vi "check out and in tracking spot null tester.vi"(0 "N spot tracker in":T1, 1 "set state?":bool, 5 "tracking state in":T2={"x state"={"pos estimate"=0.0, "v estimate"=0.0, "weighted position error sum"=0.0, "photon count"=0, "transmit tick count"=0, "axis number"=0, "px (levels^2)"=0.0, "pxv (levels^2/ticks)"=0.0, "pv (levels^2/ticks^2)"=0.0, "vel diff (levels^2/ticks^3)"=0.0, "gx"=0.0, "rtwiddle"=0.0, "photon count ch0"=0, "photon count ch1"=0, "Dx - for pos only k-f"=0.0}, "y state"={"pos estimate"=0.0, "v estimate"=0.0, "weighted position error sum"=0.0, "photon count"=0, "transmit tick count"=0, "axis number"=1, "px (levels^2)"=0.0, "pxv (levels^2/ticks)"=0.0, "pv (levels^2/ticks^2)"=0.0, "vel diff (levels^2/ticks^3)"=0.0, "gx"=0.0, "rtwiddle"=0.0, "photon count ch0"=0, "photon count ch1"=0, "Dx - for pos only k-f"=0.0}, "z state"={"pos estimate"=0.0, "v estimate"=0.0, "weighted position error sum"=0.0, "photon count"=0, "transmit tick count"=0, "axis number"=2, "px (levels^2)"=0.0, "pxv (levels^2/ticks)"=0.0, "pv (levels^2/ticks^2)"=0.0, "vel diff (levels^2/ticks^3)"=0.0, "gx"=0.0, "rtwiddle"=0.0, "photon count ch0"=0, "photon count ch1"=0, "Dx - for pos only k-f"=0.0}}, 7 "new circle":bool, 9 "permission to swap states":bool, 11 "set state value":T2={"x state"={"pos estimate"=0.0, "v estimate"=0.0, "weighted position error sum"=0.0, "photon count"=0, "transmit tick count"=0, "axis number"=0, "px (levels^2)"=0.0, "pxv (levels^2/ticks)"=0.0, "pv (levels^2/ticks^2)"=0.0, "vel diff (levels^2/ticks^3)"=0.0, "gx"=0.0, "rtwiddle"=0.0, "photon count ch0"=0, "photon count ch1"=0, "Dx - for pos only k-f"=0.0}, "y state"={"pos estimate"=0.0, "v estimate"=0.0, "weighted position error sum"=0.0, "photon count"=0, "transmit tick count"=0, "axis number"=1, "px (levels^2)"=0.0, "pxv (levels^2/ticks)"=0.0, "pv (levels^2/ticks^2)"=0.0, "vel diff (levels^2/ticks^3)"=0.0, "gx"=0.0, "rtwiddle"=0.0, "photon count ch0"=0, "photon count ch1"=0, "Dx - for pos only k-f"=0.0}, "z state"={"pos estimate"=0.0, "v estimate"=0.0, "weighted position error sum"=0.0, "photon count"=0, "transmit tick count"=0, "axis number"=2, "px (levels^2)"=0.0, "pxv (levels^2/ticks)"=0.0, "pv (levels^2/ticks^2)"=0.0, "vel diff (levels^2/ticks^3)"=0.0, "gx"=0.0, "rtwiddle"=0.0, "photon count ch0"=0, "photon count ch1"=0, "Dx - for pos only k-f"=0.0}}, 12 "state number to set":u8) -> (4 "N spot tracker out":T1, 6 "tracking state out":T2={"x state"={"pos estimate"=0.0, "v estimate"=0.0, "weighted position error sum"=0.0, "photon count"=0, "transmit tick count"=0, "axis number"=0, "px (levels^2)"=0.0, "pxv (levels^2/ticks)"=0.0, "pv (levels^2/ticks^2)"=0.0, "vel diff (levels^2/ticks^3)"=0.0, "gx"=0.0, "rtwiddle"=0.0, "photon count ch0"=0, "photon count ch1"=0, "Dx - for pos only k-f"=0.0}, "y state"={"pos estimate"=0.0, "v estimate"=0.0, "weighted position error sum"=0.0, "photon count"=0, "transmit tick count"=0, "axis number"=1, "px (levels^2)"=0.0, "pxv (levels^2/ticks)"=0.0, "pv (levels^2/ticks^2)"=0.0, "vel diff (levels^2/ticks^3)"=0.0, "gx"=0.0, "rtwiddle"=0.0, "photon count ch0"=0, "photon count ch1"=0, "Dx - for pos only k-f"=0.0}, "z state"={"pos estimate"=0.0, "v estimate"=0.0, "weighted position error sum"=0.0, "photon count"=0, "transmit tick count"=0, "axis number"=2, "px (levels^2)"=0.0, "pxv (levels^2/ticks)"=0.0, "pv (levels^2/ticks^2)"=0.0, "vel diff (levels^2/ticks^3)"=0.0, "gx"=0.0, "rtwiddle"=0.0, "photon count ch0"=0, "photon count ch1"=0, "Dx - for pos only k-f"=0.0}}, 8 "checked out state number":u8, 10 "use photons to track":bool)   [LabVIEW 2010]
uses:
  kalman 3-axis state.ctl
  integrating single axis kalman state.ctl
  kalman N spot state.ctl
panel:
  in  "tracking?":bool=TRUE
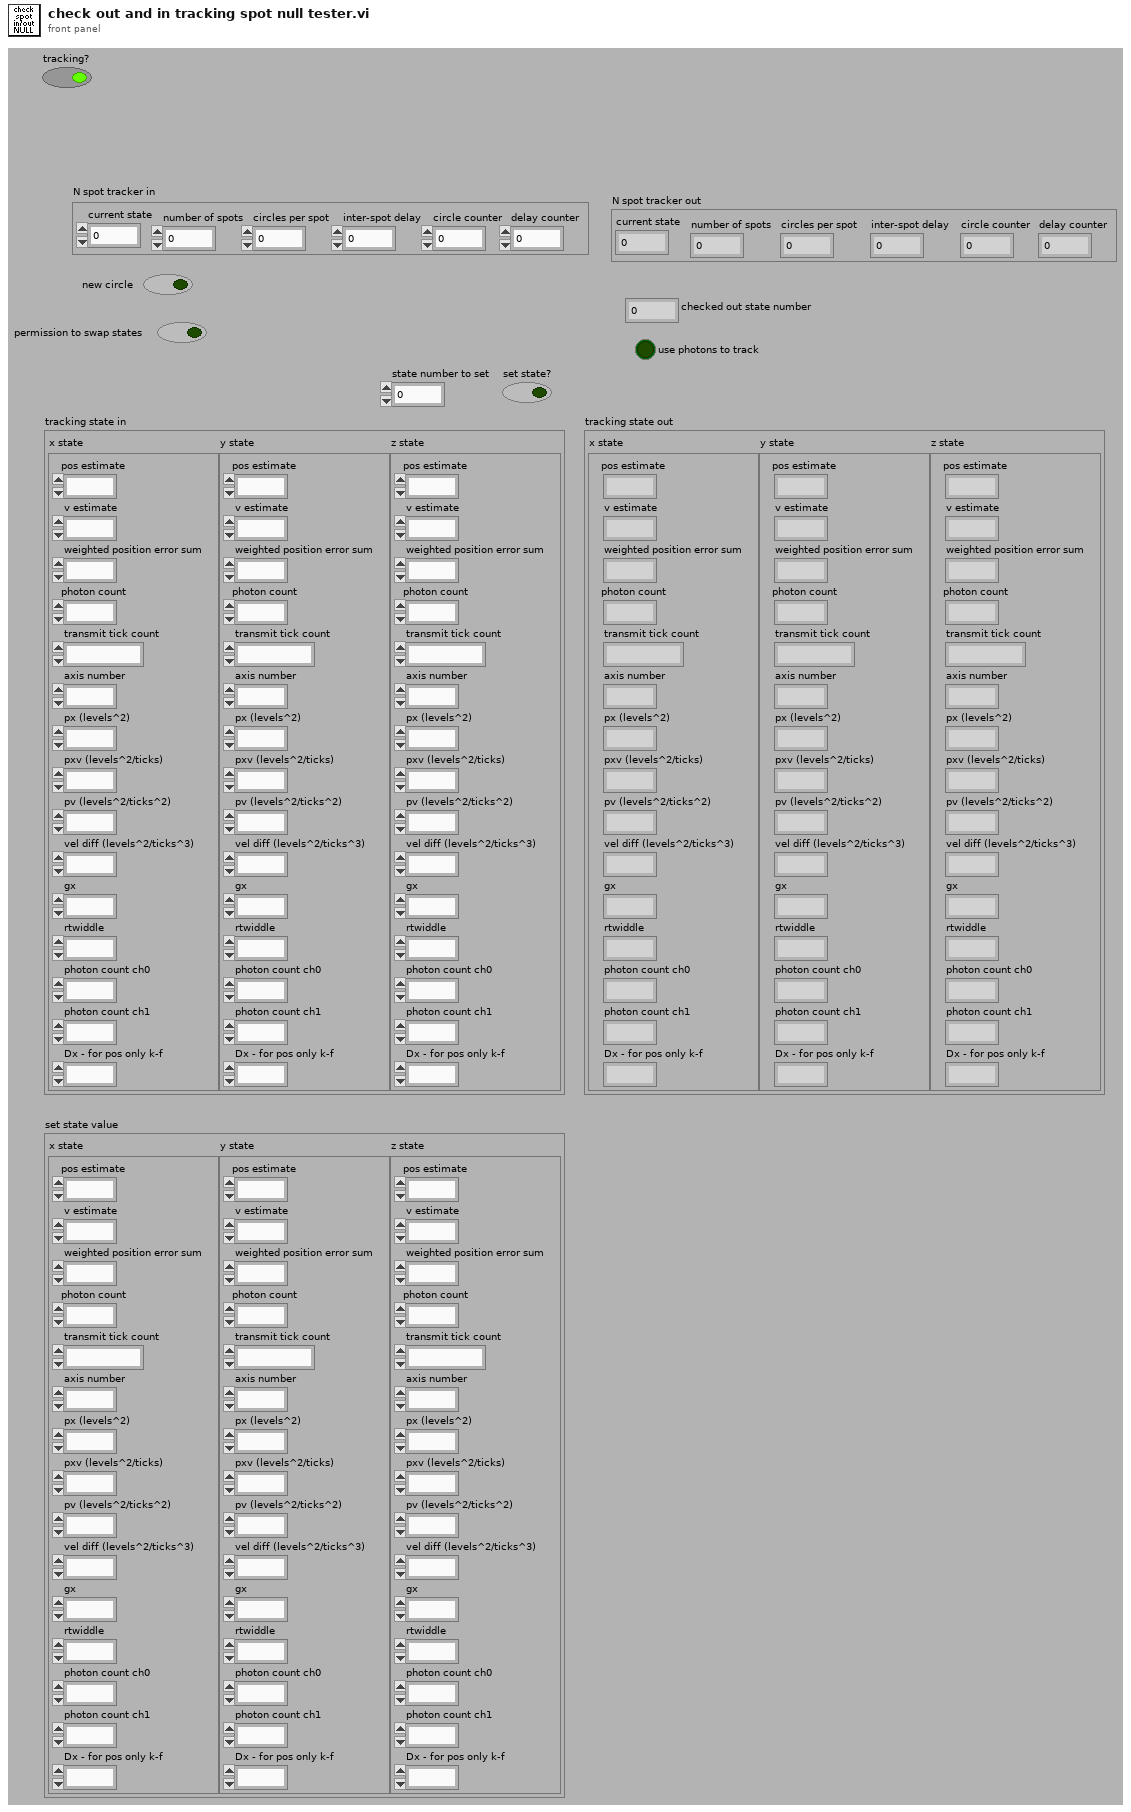
[diagram p1: front panel]
types:
  T1 = typedef "kalman N spot state.ctl" = cluster{"current state":u8, "number of spots":u8, "circles per spot":u8, "inter-spot delay":u8, "circle counter":u8, "delay counter":u8}
  T2 = typedef "kalman 3-axis state.ctl" = cluster{"x state":T3, "y state":T3, "z state":T3}
  T3 = typedef "integrating single axis kalman state.ctl" = cluster{"pos estimate":fxp<+/-,32,16>, "v estimate":fxp<+/-,16,0>, "weighted position error sum":fxp<+/-,32,32>, "photon count":u32, "transmit tick count":u32, "axis number":u8, "px (levels^2)":fxp<+,32,19>, "pxv (levels^2/ticks)":fxp<+,32,2>, "pv (levels^2/ticks^2)":fxp<+,32,-14>, "vel diff (levels^2/ticks^3)":fxp<+,24,-22>, "gx":fxp<+,16,8>, "rtwiddle":fxp<+,16,26>, "photon count ch0":u32, "photon count ch1":u32, "Dx - for pos only k-f":fxp<+,32,19>}
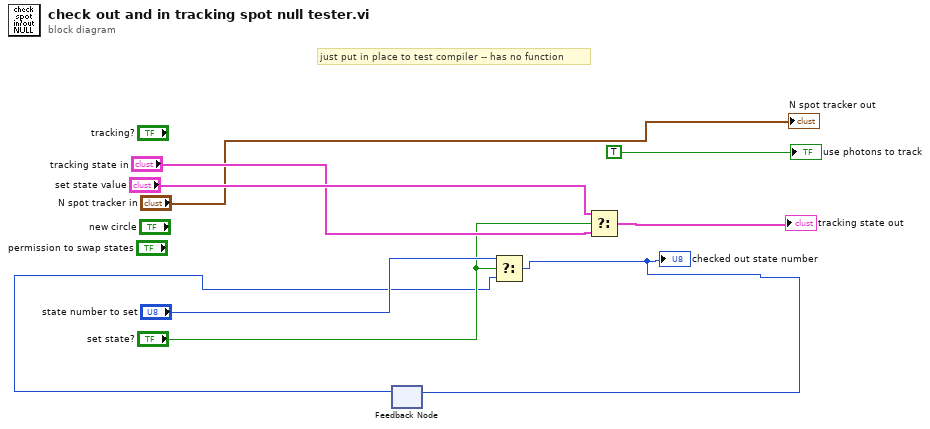
[diagram p0: block diagram]
diagram:
  # "just put in place to test compiler -- has no function"
  n1 = feedback #1() -> (w1:u8)  [unwired: 1 in]
  n2 = Select(t="state number to set", s="set state?", f=w1) -> (s? t:f=w2:u8)
  "checked out state number" <- w2
  n3 = feedback-in #1(w2) -> ()
  n4 = Select(t="set state value", s="set state?", f="tracking state in") -> (s? t:f=→"tracking state out":T2)
  "N spot tracker out" <- "N spot tracker in"
  "use photons to track" <- TRUE ("use photons to track")
